vi "Binary Stream Writer.vi"(8 "error in (no error)":errorcluster, 9 ".NET AdsBinaryWriter refnum":refnum<k24>, 10 "Value":variant, 11 "TwinCAT ADS in":refnum<class "TwinCAT ADS.lvclass">) -> (0 "error out":errorcluster, 1 ".NET AdsBinaryWriter refnum":refnum<k24>, 3 "TwinCAT ADS out":refnum<class "TwinCAT ADS.lvclass">, 4 "Length":i64)   [LabVIEW 2018, in "TwinCAT ADS.lvclass"]
uses:
  TwinCAT ADS.lvclass
  TwinCAT.Ads
  <vilib>/Utility/Data Type/NI_Data Type.lvlib
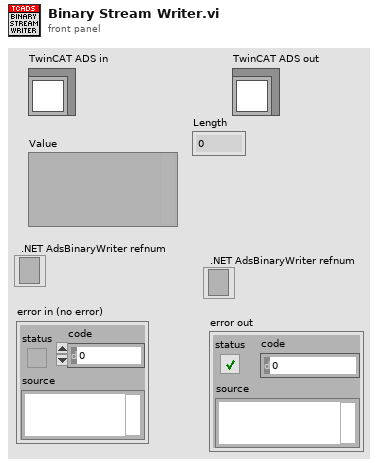
[diagram p1: front panel]
types:
  T1 = typedef "NI_Data Type.lvlib/Data Type.ctl" = enum8{"Invalid Type", "Void", "I8", "I16", "I32", "I64", "U8", "U16", "U32", "U64", "Single Float", "Double Float", "Extended Float", "Single Complex", "Double Complex", "Extended Complex", "Enum U8", "Enum U16", "Enum U32", "Enum U64", "Single Float With Unit", "Double Float With Unit", "Extended Float With Unit", "Single Complex with Unit", "Double Complex with Unit", "Extended Complex with Unit", "Boolean", "String", "Path", "Picture", "Tag", "Array", "Cluster", "Variant", "LV Variant", "Waveform", "Timestamp", "Digital Waveform", "Digital Data", "ExpressData", "Refnum", "External Data", "VI", "Poly VI", "LabVIEW Class Instance", "Fixed Point"}
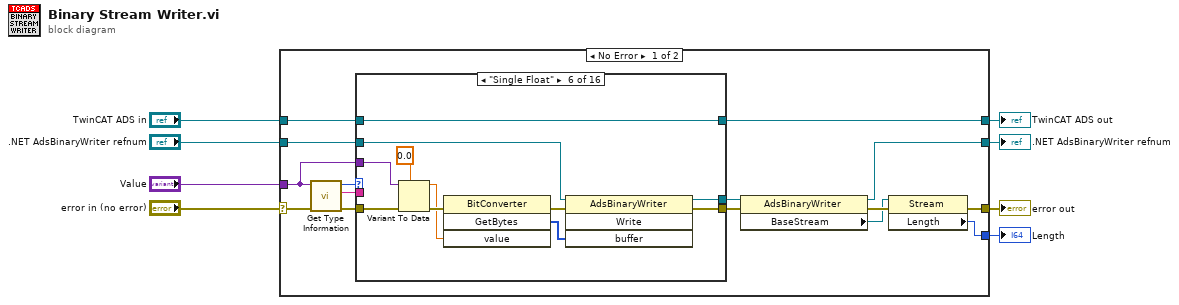
[diagram p0: block diagram]
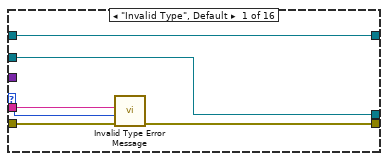
[diagram p2: hidden frame]
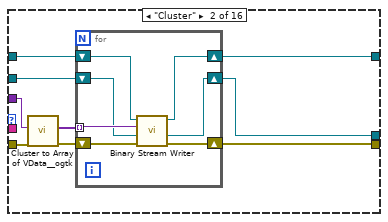
[diagram p3: hidden frame]
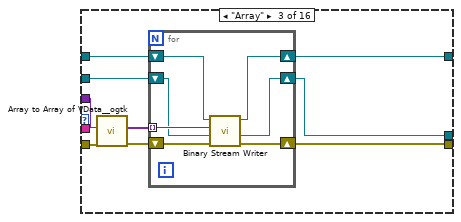
[diagram p4: hidden frame]
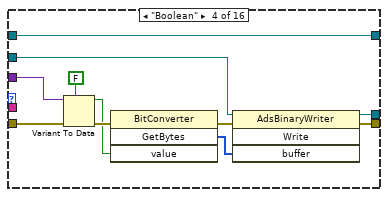
[diagram p5: hidden frame]
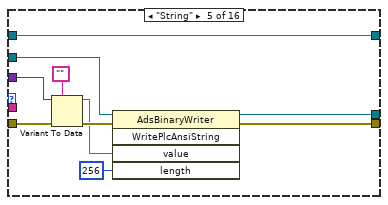
[diagram p6: hidden frame]
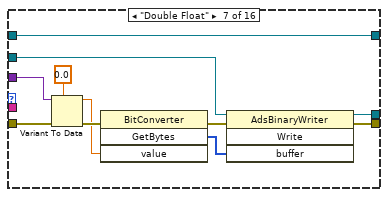
[diagram p7: hidden frame]
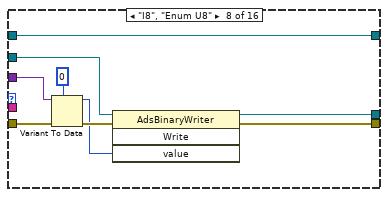
[diagram p8: hidden frame]
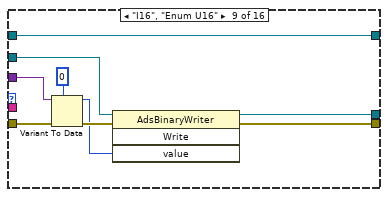
[diagram p9: hidden frame]
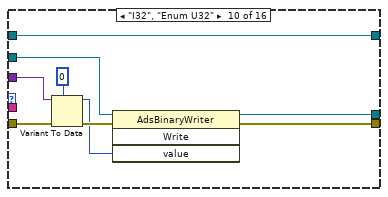
[diagram p10: hidden frame]
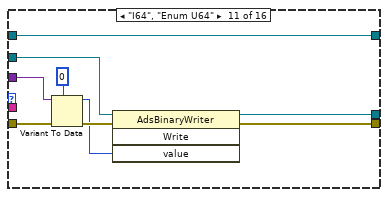
[diagram p11: hidden frame]
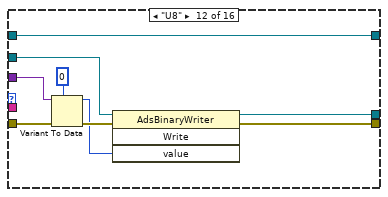
[diagram p12: hidden frame]
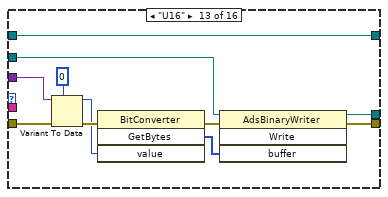
[diagram p13: hidden frame]
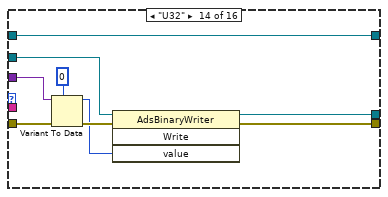
[diagram p14: hidden frame]
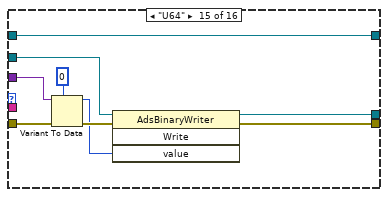
[diagram p15: hidden frame]
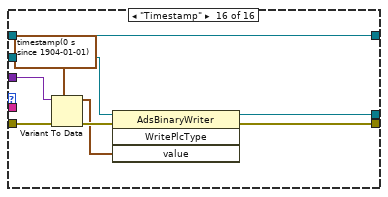
[diagram p16: hidden frame]
diagram:
  n1 = case shown="No Error" "error in (no error)" {
    selector: "error in (no error)" -> [w17 w189]
    tunnel: "Value" -> [w21 _]
    tunnel: ".NET AdsBinaryWriter refnum" -> [w20 w188]
    tunnel: [w11 w189] -> w6
    tunnel: "TwinCAT ADS in" -> [w19 w190]
    tunnel: [w18 w190] -> w4
    tunnel: [w10 w188] -> w2
    tunnel: [w9 _] -> w1
    frame No Error {
      n2 = call <vilib>:"Get Type Information.vi"("error in (no error)"=w17, "Variant"=w21) -> ("error out"=w23:errorcluster, "Name"=w16:string, "Type"=w22:T1)  [unwired: 5 in, 2 out]
      n3 = case shown="\"Single Float\"" w22 {
        selector: w22 -> [w24 _ _ _ _ _ _ _ _ _ _ _ _ _ _ _]
        tunnel: w21 -> [_ w37 w47 w72 w82 w93 w104 w113 w122 w131 w140 w149 w160 w169 w178 w187]
        tunnel: w20 -> [w28 w33 w53 w67 w80 w85 w103 w111 w120 w129 w138 w147 w152 w167 w176 w185]
        tunnel: [w26 w35 w54 w70 w78 w83 w102 w110 w119 w128 w137 w146 w150 w166 w175 w184] -> w15
        tunnel: w23 -> [w27 w38 w50 w66 w75 w90 w98 w105 w114 w123 w132 w141 w157 w161 w170 w181]
        tunnel: w19 -> [w29 w32 w52 w69 w74 w91 w100 w107 w116 w125 w134 w143 w158 w163 w172 w183]
        tunnel: [w29 w31 w51 w69 w74 w91 w100 w107 w116 w125 w134 w143 w158 w163 w172 w183] -> w18
        tunnel: [w28 w30 w46 w68 w73 w84 w99 w106 w115 w124 w133 w142 w151 w162 w171 w182] -> w14
        tunnel: w16 -> [w25 _ _ _ _ _ _ _ _ _ _ _ _ _ _ _]
        frame "Invalid Type", Default {
          n4 = call "Invalid Type Error Message.vi"("error in (no error)"=w27, "Type"=w24, "Name"=w25) -> ("error out"=w26:errorcluster)  [unwired: 7 in, 1 out]
        }
        frame "Cluster" {
          n5 = call <userlib>:"Cluster to Array of VData__ogtk.vi"("error in (no error)"=w38, "Cluster"=w37) -> ("error out"=w36:errorcluster, "Array of VData"=w34:variant[])  [unwired: 8 in]
          n6 = for {
            shift-right: [w44] -> w35
            shift-left: w36 -> [w45]
            tunnel: w34 -> [w41] mode=indexing
            shift-right: [w42] -> w31
            shift-left: w32 -> [w43]
            shift-right: [w39] -> w30
            shift-left: w33 -> [w40]
            n7 = call "Binary Stream Writer.vi"("error in (no error)"=w45, ".NET AdsBinaryWriter refnum"=w40, "Value"=w41, "TwinCAT ADS in"=w43) -> ("error out"=w44:errorcluster, ".NET AdsBinaryWriter refnum"=w39:refnum<k24>, "TwinCAT ADS out"=w42:refnum<class "TwinCAT ADS.lvclass">)  [unwired: 4 in, 1 out]
          }
        }
        frame "Array" {
          n8 = call <userlib>:"Array to Array of VData__ogtk.vi"("error in (no error)"=w50, "MultiD Array"=w47) -> ("error out"=w49:errorcluster, "1D Array of Variants"=w48:variant[])  [unwired: 8 in]
          n9 = for {
            shift-right: [w60] -> w54
            shift-left: w49 -> [w61]
            tunnel: w48 -> [w57] mode=indexing
            shift-right: [w58] -> w51
            shift-left: w52 -> [w59]
            shift-right: [w55] -> w46
            shift-left: w53 -> [w56]
            n10 = call "Binary Stream Writer.vi"("error in (no error)"=w61, ".NET AdsBinaryWriter refnum"=w56, "Value"=w57, "TwinCAT ADS in"=w59) -> ("error out"=w60:errorcluster, ".NET AdsBinaryWriter refnum"=w55:refnum<k24>, "TwinCAT ADS out"=w58:refnum<class "TwinCAT ADS.lvclass">)  [unwired: 4 in, 1 out]
          }
        }
        frame "Boolean" {
          n11 = Variant To Data(error in=w66, type=FALSE, Variant=w72) -> (data=w63:bool, error out=w64:errorcluster)
          n12 = invoke class="BitConverter" method="GetBytes"(error in=w64, "value"=w63) -> (error out=w65:errorcluster, "GetBytes"=w62:u8[])  [unwired: 2 in, 2 out]
          n13 = invoke class="AdsBinaryWriter" method="Write"(reference=w67, error in=w65, "buffer"=w62) -> (reference out=w68:refnum<k24>, error out=w70:errorcluster)  [unwired: 1 in, 2 out]
        }
        frame "String" {
          n14 = Variant To Data(error in=w75, type="", Variant=w82) -> (data=w79:string, error out=w81:errorcluster)
          n15 = invoke class="AdsBinaryWriter" method="WritePlcAnsiString"(reference=w80, error in=w81, "value"=w79, "length"=256) -> (reference out=w73:refnum<k24>, error out=w78:errorcluster)  [unwired: 1 in, 3 out]
        }
        frame "Single Float" {
          n16 = Variant To Data(error in=w90, type=sgl 0.0 ("value"), Variant=w93) -> (data=w86:sgl, error out=w87:errorcluster)
          n17 = invoke class="BitConverter" method="GetBytes"(error in=w87, "value"=w86) -> (error out=w89:errorcluster, "GetBytes"=w88:u8[])  [unwired: 2 in, 2 out]
          n18 = invoke class="AdsBinaryWriter" method="Write"(reference=w85, error in=w89, "buffer"=w88) -> (reference out=w84:refnum<k24>, error out=w83:errorcluster)  [unwired: 1 in, 2 out]
        }
        frame "Double Float" {
          n19 = Variant To Data(error in=w98, type=0.0 ("value"), Variant=w104) -> (data=w94:dbl, error out=w97:errorcluster)
          n20 = invoke class="BitConverter" method="GetBytes"(error in=w97, "value"=w94) -> (error out=w96:errorcluster, "GetBytes"=w95:u8[])  [unwired: 2 in, 2 out]
          n21 = invoke class="AdsBinaryWriter" method="Write"(reference=w103, error in=w96, "buffer"=w95) -> (reference out=w99:refnum<k24>, error out=w102:errorcluster)  [unwired: 1 in, 2 out]
        }
        frame "I8", "Enum U8" {
          n22 = Variant To Data(error in=w105, type=i8 0 ("value"), Variant=w113) -> (data=w108:i8, error out=w112:errorcluster)
          n23 = invoke class="AdsBinaryWriter" method="Write"(reference=w111, error in=w112, "value"=w108) -> (reference out=w106:refnum<k24>, error out=w110:errorcluster)  [unwired: 1 in, 2 out]
        }
        frame "I16", "Enum U16" {
          n24 = Variant To Data(error in=w114, type=i16 0 ("value"), Variant=w122) -> (data=w117:i16, error out=w121:errorcluster)
          n25 = invoke class="AdsBinaryWriter" method="Write"(reference=w120, error in=w121, "value"=w117) -> (reference out=w115:refnum<k24>, error out=w119:errorcluster)  [unwired: 1 in, 2 out]
        }
        frame "I32", "Enum U32" {
          n26 = Variant To Data(error in=w123, type=0 ("value"), Variant=w131) -> (data=w126:i32, error out=w130:errorcluster)
          n27 = invoke class="AdsBinaryWriter" method="Write"(reference=w129, error in=w130, "value"=w126) -> (reference out=w124:refnum<k24>, error out=w128:errorcluster)  [unwired: 1 in, 2 out]
        }
        frame "I64", "Enum U64" {
          n28 = Variant To Data(error in=w132, type=i64 0 ("value"), Variant=w140) -> (data=w135:i64, error out=w139:errorcluster)
          n29 = invoke class="AdsBinaryWriter" method="Write"(reference=w138, error in=w139, "value"=w135) -> (reference out=w133:refnum<k24>, error out=w137:errorcluster)  [unwired: 1 in, 2 out]
        }
        frame "U8" {
          n30 = Variant To Data(error in=w141, type=u8 0 ("value"), Variant=w149) -> (data=w144:u8, error out=w148:errorcluster)
          n31 = invoke class="AdsBinaryWriter" method="Write"(reference=w147, error in=w148, "value"=w144) -> (reference out=w142:refnum<k24>, error out=w146:errorcluster)  [unwired: 1 in, 2 out]
        }
        frame "U16" {
          n32 = Variant To Data(error in=w157, type=u16 0 ("value"), Variant=w160) -> (data=w153:u16, error out=w154:errorcluster)
          n33 = invoke class="BitConverter" method="GetBytes"(error in=w154, "value"=w153) -> (error out=w155:errorcluster, "GetBytes"=w156:u8[])  [unwired: 2 in, 2 out]
          n34 = invoke class="AdsBinaryWriter" method="Write"(reference=w152, error in=w155, "buffer"=w156) -> (reference out=w151:refnum<k24>, error out=w150:errorcluster)  [unwired: 1 in, 2 out]
        }
        frame "U32" {
          n35 = Variant To Data(error in=w161, type=u32 0 ("value"), Variant=w169) -> (data=w164:u32, error out=w168:errorcluster)
          n36 = invoke class="AdsBinaryWriter" method="Write"(reference=w167, error in=w168, "value"=w164) -> (reference out=w162:refnum<k24>, error out=w166:errorcluster)  [unwired: 1 in, 2 out]
        }
        frame "U64" {
          n37 = Variant To Data(error in=w170, type=u64 0 ("value"), Variant=w178) -> (data=w173:u64, error out=w177:errorcluster)
          n38 = invoke class="AdsBinaryWriter" method="Write"(reference=w176, error in=w177, "value"=w173) -> (reference out=w171:refnum<k24>, error out=w175:errorcluster)  [unwired: 1 in, 2 out]
        }
        frame "Timestamp" {
          n39 = Variant To Data(error in=w181, type=timestamp(0 s since 1904-01-01) ("value"), Variant=w187) -> (data=w179:timestamp, error out=w186:errorcluster)
          n40 = invoke class="AdsBinaryWriter" method="WritePlcType"(reference=w185, error in=w186, "value"=w179) -> (reference out=w182:refnum<k24>, error out=w184:errorcluster)  [unwired: 1 in, 2 out]
        }
      }
      n41 = property class="AdsBinaryWriter"(reference=w14, error in=w15) -> (reference out=w10:refnum<k24>, error out=w13:errorcluster, "BaseStream"=w12:refnum<k24>)
      n42 = property class="Stream"(reference=w12, error in=w13) -> (error out=w11:errorcluster, "Length"=w9:i64)  [unwired: 1 out]
    }
    frame Error {
    }
  }
  "error out" <- w6
  "TwinCAT ADS out" <- w4
  ".NET AdsBinaryWriter refnum" <- w2
  "Length" <- w1
